vi "mtg reader demo.vi"() -> ()   [LabVIEW 2025]
uses:
  mtg reader - globals.vi
panel:
  out "time at cursor":dbl format="%<%H:%M:%S\n%Y/%m/%d>T"
  out "session folders":string[][](table)
  out "session files":string[][](table)
  in  "stop":bool
  in  "session file selection":i32(slide) min=0 max=138
  out "1 hour chart":dbl[][](graph)
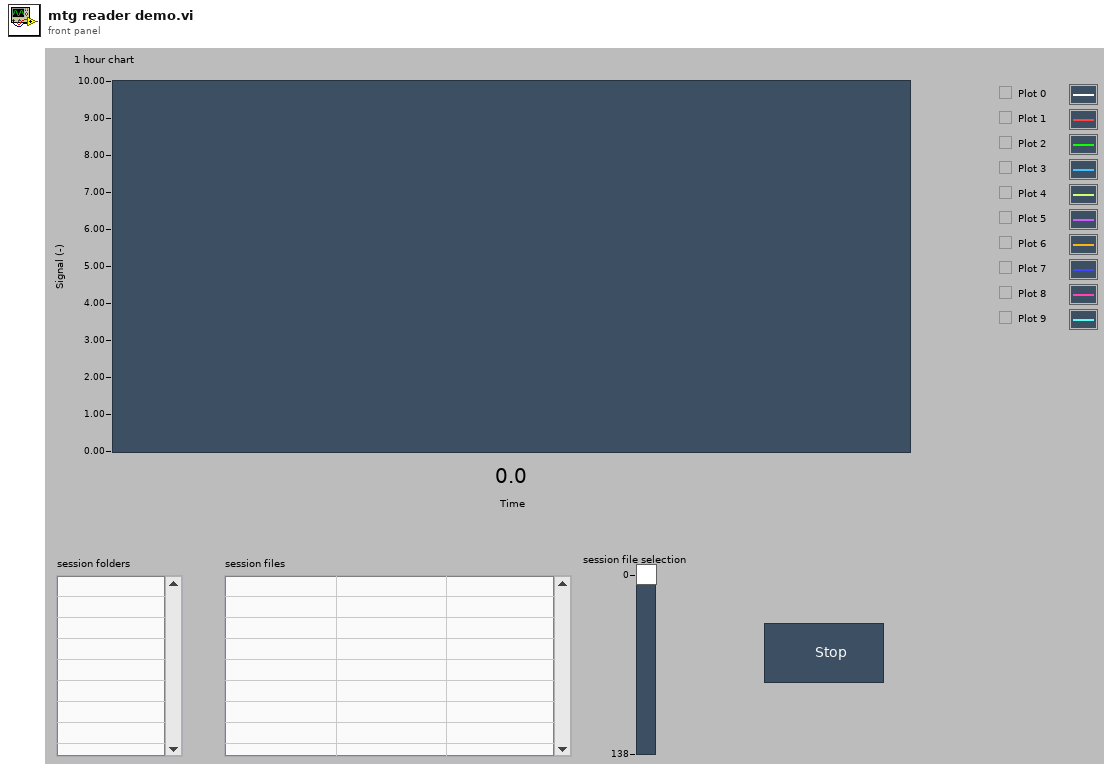
[diagram p1: front panel]
types:
  T1 = cluster{"path calling vi":path, "base directory":string, "session folders table":refnum<vi>}
  T2 = typedef "LVRowAndColumnTypeDef.ctl" = cluster{"Row":i32, "Column":i32}
  T3 = typedef "LVPoint32TypeDef.ctl" = cluster{"Horizontal":i32, "Vertical":i32}
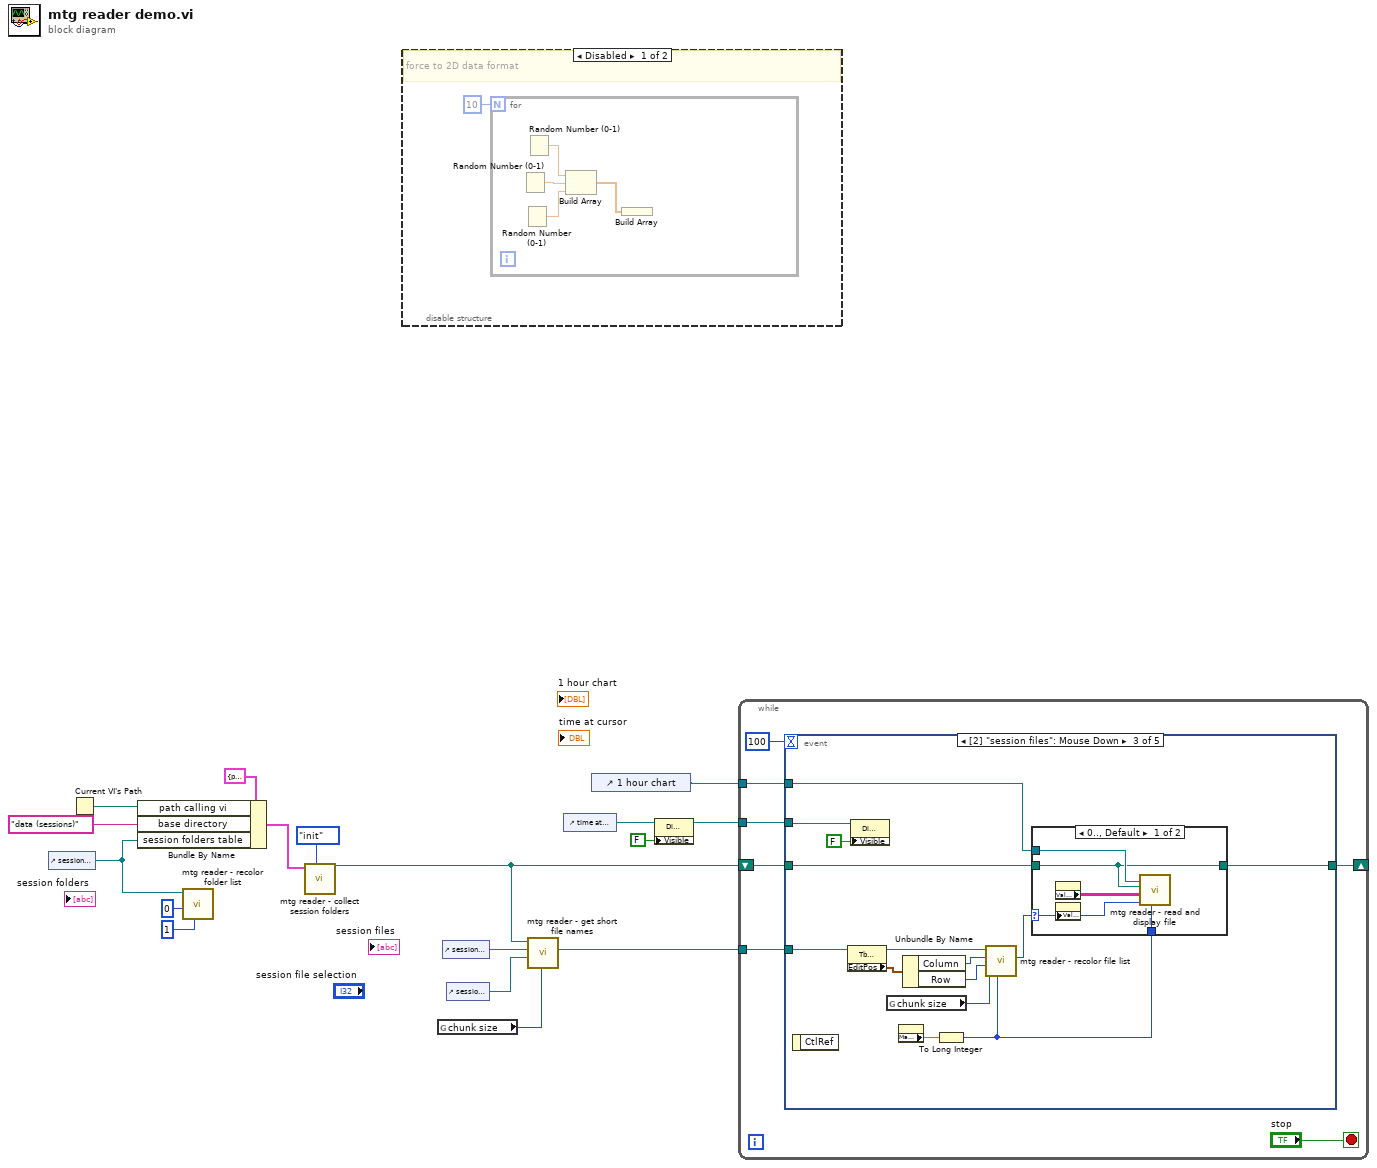
[diagram p0: block diagram]
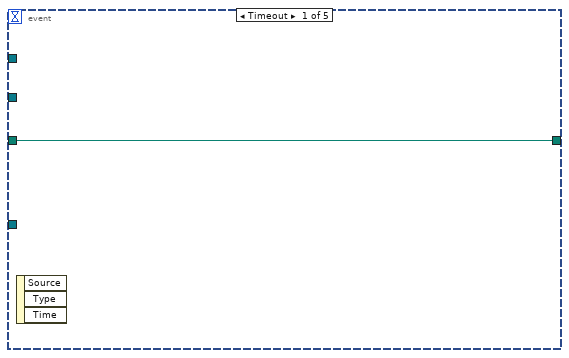
[diagram p2: hidden frame]
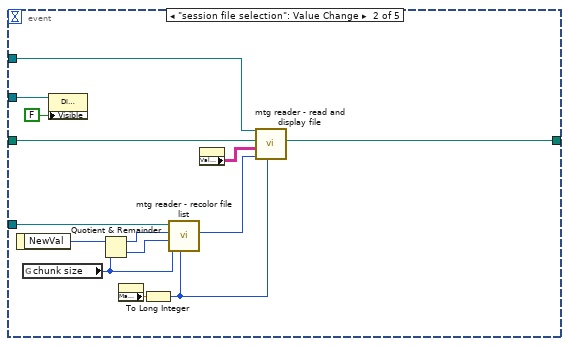
[diagram p3: hidden frame]
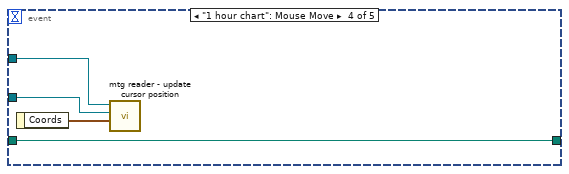
[diagram p5: hidden frame]
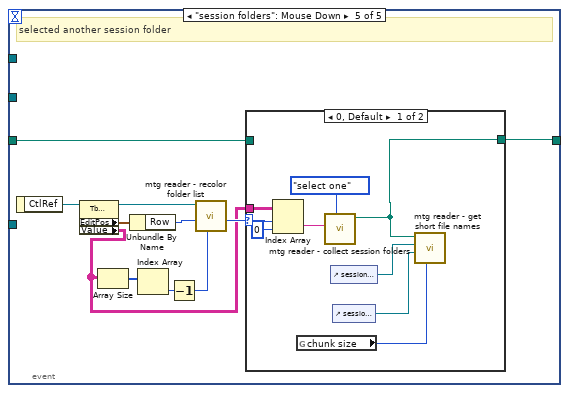
[diagram p6: hidden frame]
diagram:
  n1 = control-ref of="session folders"() -> (w4:refnum<vi>)
  n2 = Current VI's Path() -> (path=w11:path)
  n3 = Bundle By Name(cluster=T1 {"path calling vi"=path "H:/LabVIEW/_tools/mtg/mtg reader demo.vi", "base directory"="data (sessions)", "session folders table"=refnum} ("config"), "path calling vi"=w11, "base directory"="data (sessions)", "session folders table"=w4) -> (w9:T1)
  n4 = call "mtg reader - recolor folder list.vi"("max index"=1, "Row in"=0, "table ref"=w4) -> ()  [unwired: 7 in, 2 out]
  n5 = call "mtg reader - collect session folders.vi"("action"=enum16{"init", "refresh", "select one"}."init", "config"=w9) -> ("selected session folder"=w17:path)  [unwired: 8 in, 1 out]
  n6 = disable-structure shown="Disabled" {
    frame Disabled {
      # "force to 2D data format"
      n7 = for {
        N: 10 -> [_]
        n8 = Random Number (0-1)() -> (number: 0 to 1=w21:dbl)
        n9 = Random Number (0-1)() -> (number: 0 to 1=w20:dbl)
        n10 = Random Number (0-1)() -> (number: 0 to 1=w22:dbl)
        n11 = Build Array(w22, w21, w20) -> (w19:dbl[])
        n12 = Build Array(w19) -> ()  [unwired: 1 out]
      }
    }
    frame Enabled {
    }
  }
  n13 = global read "mtg reader - globals.vi" "chunk size"() -> (w1:i32)
  n14 = control-ref of="session files"() -> (w7:refnum<vi>)
  n15 = control-ref of="session file selection"() -> (w6:refnum<vi>)
  n16 = call "mtg reader - get short file names.vi"("rowsize"=w1, "session file selection"=w6, "session files in"=w7, "data (session)"=w17) -> ("session files out"=w2:refnum<vi>)  [unwired: 7 in]
  n17 = control-ref of="time at cursor"() -> (w15:refnum<vi>)
  n18 = control-ref of="1 hour chart"() -> (w16:refnum<vi>)
  n19 = property class="DigNum (strict)"(reference=w15, "Visible"=FALSE) -> (reference out=w14:refnum<vi>)  [unwired: 1 in, 1 out]
  n20 = while {
    tunnel: w2 -> [w27]
    tunnel: w16 -> [w26]
    tunnel: w14 -> [w24]
    shift-right: [w23] -> _
    shift-left: w17 -> [w25]
    stop <- "stop" stop-if-true
    n21 = event shown="[2] \"session files\": Mouse Down" {
      selector: _ -> [_ _ _ _ _]
      dyn-events: _ -> [_ _ _ _ _]
      timeout: 100 -> [_ _ _ _ _]
      tunnel: w27 -> [_ w43 w47 _ _]
      tunnel: w26 -> [_ w40 w53 w68 _]
      tunnel: w25 -> [w30 w39 w52 w65 w70]
      tunnel: w24 -> [_ w35 w50 w66 _]
      tunnel: [w30 w32 w46 w65 w69] -> w23
      event Timeout {
        n22 = event-data() -> ()  [unwired: 1 in, 3 out]
      }
      event "session file selection": Value Change {
        n23 = event-data() -> ("NewVal"=w44:i32)  [unwired: 1 in]
        n24 = global read "mtg reader - globals.vi" "chunk size"() -> (w31:i32)
        n25 = property class="DigNum (strict)"(reference=w35, "Visible"=FALSE) -> ()  [unwired: 1 in, 2 out]
        n26 = Quotient & Remainder(x=w44, y=w31) -> (x-y*floor(x/y)=w42:i32, floor(x/y)=w41:i32)
        n27 = property on="session file selection" class="Slide (strict)"() -> ("Maximum"=w34:dbl)  [unwired: 2 in, 2 out]
        n28 = To Long Integer(number=w34) -> (32bit integer=w33:i32)
        n29 = call "mtg reader - recolor file list.vi"("max index"=w33, "rowsize"=w31, "Row"=w41, "Column"=w42, "table ref"=w43) -> ("slider pos"=w37:i32)  [unwired: 5 in, 1 out]
        n30 = property on="session files" class="Tbl (strict)"() -> ("Value"=w38:string[][])  [unwired: 2 in, 2 out]
        n31 = call "mtg reader - read and display file.vi"("max index"=w33, "index"=w37, "session file"=w38, "data (sessions folder)"=w39, "WaveformChart in"=w40) -> ("data (sessions folder) out"=w32:path)  [unwired: 5 in, 1 out]
      }
      event "session files": Mouse Down {
        n32 = event-data() -> ()  [unwired: 1 in, 1 out]
        n33 = property class="Tbl (strict)"(reference=w47) -> (reference out=w58:refnum<vi>, "EditPos"=w57:T2)  [unwired: 1 in, 1 out]
        n34 = property class="DigNum (strict)"(reference=w50, "Visible"=FALSE) -> ()  [unwired: 1 in, 2 out]
        n35 = global read "mtg reader - globals.vi" "chunk size"() -> (w45:i32)
        n36 = property on="session file selection" class="Slide (strict)"() -> ("Maximum"=w49:dbl)  [unwired: 2 in, 2 out]
        n37 = Unbundle By Name(w57) -> ("Column"=w56:i32, "Row"=w55:i32)
        n38 = To Long Integer(number=w49) -> (32bit integer=w48:i32)
        n39 = call "mtg reader - recolor file list.vi"("max index"=w48, "rowsize"=w45, "Row"=w55, "Column"=w56, "table ref"=w58) -> ("slider pos"=w54:i32)  [unwired: 5 in, 1 out]
        n40 = case shown="0.., Default" w54 {
          selector: w54 -> [w61 _]
          tunnel: w53 -> [w63 _]
          tunnel: w52 -> [w59 w64]
          tunnel: w48 -> [w62 _]
          tunnel: [w59 w64] -> w46
          frame 0.., Default {
            n41 = property on="session files" class="Tbl (strict)"() -> ("Value"=w60:string[][])  [unwired: 2 in, 2 out]
            n42 = property on="session file selection" class="Slide (strict)"("Value"=w61) -> ()  [unwired: 2 in, 2 out]
            n43 = call "mtg reader - read and display file.vi"("max index"=w62, "index"=w61, "session file"=w60, "data (sessions folder)"=w59, "WaveformChart in"=w63) -> ()  [unwired: 5 in, 2 out]
          }
          frame ..-1 {
          }
        }
      }
      event "1 hour chart": Mouse Move {
        n44 = event-data() -> ("Coords"=w67:T3)  [unwired: 1 in]
        n45 = call "mtg reader - update cursor position.vi"("Coords"=w67, "time at cursor"=w66, "WaveformChart in"=w68) -> ()  [unwired: 9 in]
      }
      event "session folders": Mouse Down {
        # "selected another session folder"
        n46 = event-data() -> ("CtlRef"=w78:refnum<vi>)  [unwired: 1 in]
        n47 = property class="Tbl (strict)"(reference=w78) -> (reference out=w76:refnum<vi>, "EditPos"=w79:T2, "Value"=w71:string[][])  [unwired: 1 in, 1 out]
        n48 = Array Size(array=w71) -> (size(s)=w75:i32[])
        n49 = Unbundle By Name(w79) -> ("Row"=w77:i32)
        n50 = Index Array(array=w75) -> (element=w74:i32)  [unwired: 1 in]
        n51 = Decrement(x=w74) -> (x-1=w73:i32)
        n52 = call "mtg reader - recolor folder list.vi"("max index"=w73, "Row in"=w77, "table ref"=w76) -> ("Row out"=w72:i32)  [unwired: 7 in, 1 out]
        n53 = case shown="0, Default" w72 {
          selector: w72 -> [w87 _]
          tunnel: w71 -> [w88 _]
          tunnel: w70 -> [_ w89]
          tunnel: [w83 w89] -> w69
          frame 0, Default {
            n54 = Index Array(array=w88, index (row)=w87, index (col)=0 ("disabled index (col)")) -> (element=w84:string)
            n55 = global read "mtg reader - globals.vi" "chunk size"() -> (w80:i32)
            n56 = call "mtg reader - collect session folders.vi"("action"=enum16{"init", "refresh", "select one"}."select one", "selected folder"=w84) -> ("selected session folder"=w83:path)  [unwired: 8 in, 1 out]
            n57 = control-ref of="session files"() -> (w82:refnum<vi>)
            n58 = control-ref of="session file selection"() -> (w81:refnum<vi>)
            n59 = call "mtg reader - get short file names.vi"("rowsize"=w80, "session file selection"=w81, "session files in"=w82, "data (session)"=w83) -> ()  [unwired: 7 in, 1 out]
          }
          frame -1 {
          }
        }
      }
    }
  }
